vi "FTW-Endpoint-Ask.vi"(0 "FTW Endpoint":refnum<class "FTW-Endpoint-Notifier.lvclass">, 5 "Request Header":string, 7 "Request Body":string, 9 "Timeout":i32 format="%dmsec", 11 "error in":errorcluster) -> (4 "FTW Endpoint out":refnum<class "FTW-Endpoint-Notifier.lvclass">, 6 "Response Header":string, 8 "Response Body":string, 10 "Timed out?":bool, 14 "Roundtrip Time":dbl format="%.6fsec", 15 "error out":errorcluster)   [LabVIEW 2013, in "FTW-Actor.lvlib" / "FTW-Endpoint-Notifier.lvclass"]
uses:
  FTW-Endpoint-Notifier.lvclass
panel:
  # "Inputs"
  # "Outputs"
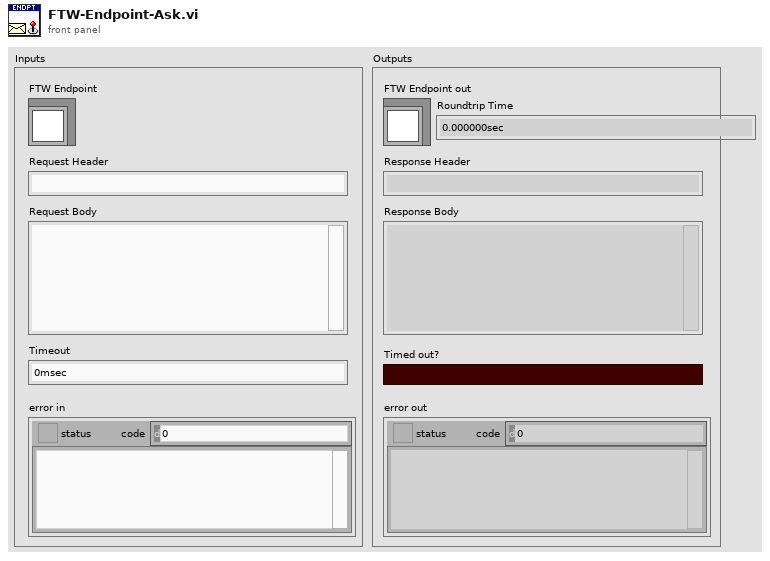
[diagram p1: front panel]
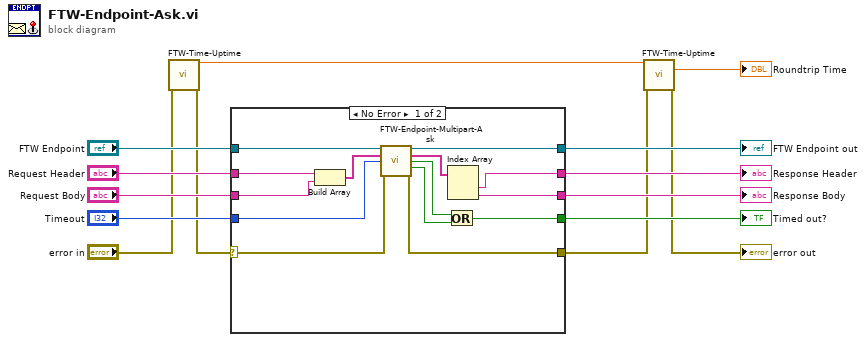
[diagram p0: block diagram]
diagram:
  n1 = call "FTW-Time-Uptime.vi"("error in"="error in") -> ("Current Uptime"=w6:dbl, "error out"=w3:errorcluster)  [unwired: 12 in, 1 out]
  n2 = case shown="No Error" w3 {
    selector: w3 -> [w24 w30]
    tunnel: [w23 w30] -> w2
    tunnel: [w25 w29] -> w13
    tunnel: "FTW Endpoint" -> [w26 w29]
    tunnel: [w18 _] -> w12
    tunnel: "Timeout" -> [w21 _]
    tunnel: "Request Header" -> [w28 _]
    tunnel: "Request Body" -> [w27 _]
    tunnel: [w16 _] -> w8
    tunnel: [w15 _] -> w7
    frame No Error {
      n3 = Build Array(w28, w27) -> (w22:string[])
      n4 = call-dynamic "FTW-Endpoint-Multipart-Ask.vi"("FTW Endpoint"=w26, "Multipart Message"=w22, "Read Timeout"=w21, "error in"=w24) -> ("FTW Endpoint out"=w25:refnum<class "FTW-Endpoint-Notifier.lvclass">, "Reply"=w17:string[], "Read Timed out?"=w20:bool, "Write Timed out?"=w19:bool, "error out"=w23:errorcluster)  [unwired: 7 in]
      n5 = Or(x=w20, y=w19) -> (x .or. y?=w18:bool)
      n6 = Index Array(array=w17) -> (element #1=w16:string, element #2=w15:string)  [unwired: 2 in]
    }
    frame Error {
    }
  }
  "FTW Endpoint out" <- w13
  "Timed out?" <- w12
  "Response Header" <- w8
  "Response Body" <- w7
  n7 = call "FTW-Time-Uptime.vi"("Previous Uptime"=w6, "error in"=w2) -> ("Elapsed Time"=→"Roundtrip Time":dbl, "error out"=→"error out":errorcluster)  [unwired: 11 in, 1 out]
